vi "OFDM-SIM去除导频.vi"(0 "经过FFT的OFDM符号":cdb[](array[numeric])) -> (1 "除去虚子载波与导频处接收的OFDM符号":cdb[](array[numeric]), 2 "信道1参数":cdb[](array[numeric]), 3 "信道2参数":cdb[](array[numeric]))   [LabVIEW 2018]
panel:
  out "大小 2":i32
  out "大小":i32
  out "插入导频处的接收信号":cdb[](array[numeric])
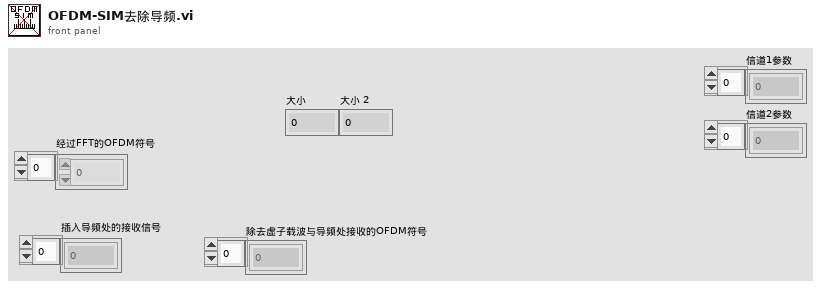
[diagram p1: front panel]
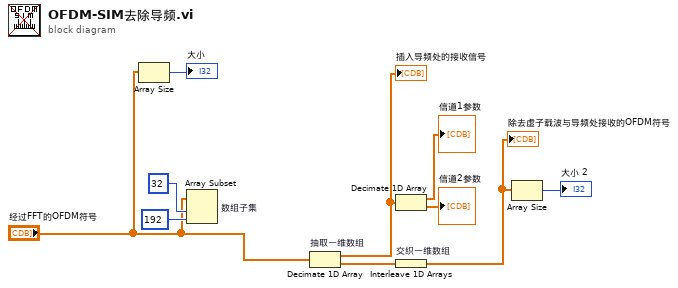
[diagram p0: block diagram]
diagram:
  n1 = Array Size(array="经过FFT的OFDM符号") -> (size(s)=→"大小":i32)
  n2 = Array Subset "数组子集"(array="经过FFT的OFDM符号", index=32 ("索引"), length=192 ("长度")) -> ()  [unwired: 1 out]
  n3 = Decimate 1D Array "抽取一维数组"("经过FFT的OFDM符号") -> (w5:cdb[], w8:cdb[])
  "插入导频处的接收信号" <- w5
  n4 = Decimate 1D Array(w5) -> (→"信道1参数":cdb[], →"信道2参数":cdb[])
  n5 = Interleave 1D Arrays "交织一维数组"(w8) -> (w2:cdb[])
  "除去虚子载波与导频处接收的OFDM符号" <- w2
  n6 = Array Size(array=w2) -> (size(s)=→"大小 2":i32)
